vi "PicoScope6000aGetStreamingLatestValues.vi"(0 "handle in":i16=16384, 1 "Polling Delays ms":T1={"Polling holdoff ms"=10, "Polling time ms"=90}, 2 "Buffer and Transfer Settings":T6={"startIndex"=0, "Samples"=1000000, "Down Sample Ratio"=1, "Down-Sample Mode"=2147483648} {"Down-Sample Mode" items=["RAW none"=2147483648, "None"=0, "Aggregate"=1, "Decimate"=2, "Average"=4]; "Down Sample Ratio" step=1; "Samples" format="%_6p"}, 3 "enabled array":i16[](array[numeric])=[1, 1, 0, 0, 0, 0, 0, 0, 0, 0], 5 "Device Info":T3, 7 "Data Pointers In":T4={"Max Buffer Pointers"=[], "Min Buffer Pointers"=[], "StreamingDataInfo"=[[{"Channel"=0, "Down-Sample Mode"=0, "PICO_DATA_TYPE"=enum."PICO_INT16_T", "Samples"=0, "bufferIndex"=0, "startIndex"=0, "overflow"=0}]]}, 9 "Buffer number":i32=1, 11 "error in (no error)":errorcluster) -> (4 "handle out":i16=16384, 8 "Data Pointers Out":T4={"Max Buffer Pointers"=[], "Min Buffer Pointers"=[], "StreamingDataInfo"=[[{"Channel"=0, "Down-Sample Mode"=0, "PICO_DATA_TYPE"=enum."PICO_INT16_T", "Samples"=0, "bufferIndex"=0, "startIndex"=0, "overflow"=0}]]}, 14 "tPicoStreamingDataTriggerInfo":T2, 15 "error out":errorcluster)   [LabVIEW 2010]
doc: "Call ps6000aGetValues to fill a single set of channel buffers."
uses:
  ps6000a.dll
  shared/PicoBuffers.ctl
  shared/Buffer and Transfer Settings.ctl
panel:
  out "No of channels":u64=2
  in  "tPicoStreamingDataInfo":T5={"Channel"=0, "Down-Sample Mode"=2147483648, "PICO_DATA_TYPE"=enum."PICO_INT16_T", "Samples"=0, "bufferIndex"=0, "startIndex"=0, "overflow"=0} {"overflow" step=1 format="%010b"; "Down-Sample Mode" items=["None"=2147483648, "Aggregate"=1, "Decimate"=2, "Average"=4]; "Channel" items=["Channel A"=0, "Channel B"=1, "Channel C"=2, "Channel D"=3, "Channel E"=4, "Channel F"=5, "Channel G"=6, "Channel H"=7, "Port 0"=128, "Port 1"=129, "Trigger AUX"=1001]; "startIndex" step=1}
  in  "Streaming Acquisition Settings":T7={"preTriggerSamples"=0, "postTriggerSamples"=1000000, "Requested sampleInterval"=1.0, "sampleIntervalTimeUnits"=3} {"sampleIntervalTimeUnits" items=["femtoseconds", "picoseconds", "nanoseconds", "microseconds", "millseconds", "seconds"]; "postTriggerSamples" format="%_6p"; "preTriggerSamples" format="%_6p"}
  # "Samples can be equal to or less\nTotal Pre and Post Trigger Samples"
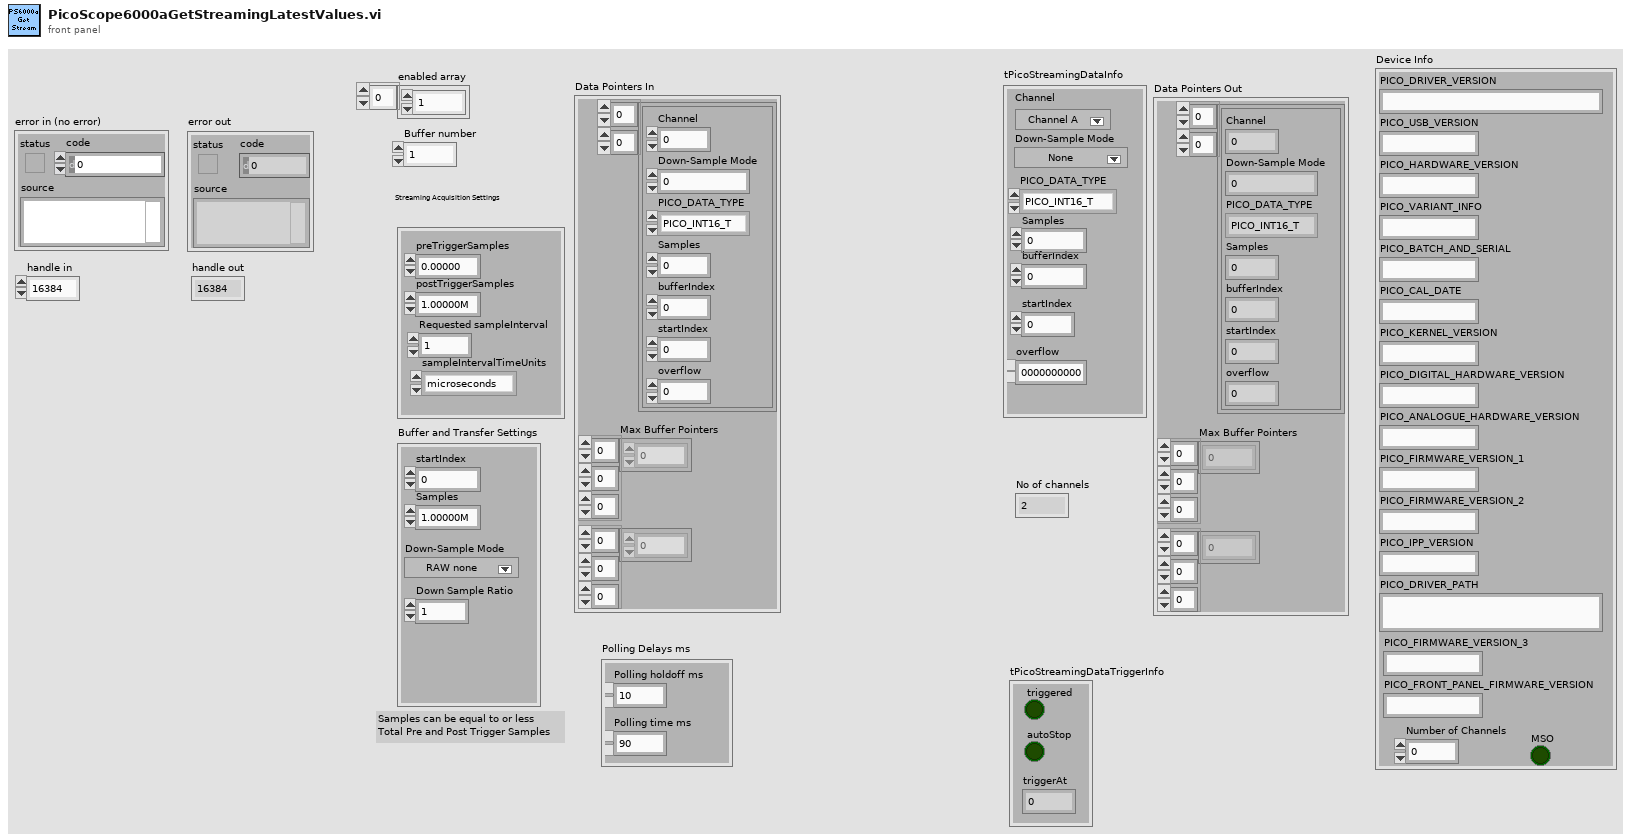
[diagram p1: front panel]
types:
  T1 = cluster{"Polling holdoff ms":u32, "Polling time ms":u32}
  T2 = cluster{"triggerAt":u64, "triggered":bool, "autoStop":bool}
  T3 = cluster{"PICO_DRIVER_VERSION":string, "PICO_USB_VERSION":string, "PICO_HARDWARE_VERSION":string, "PICO_VARIANT_INFO":string, "PICO_BATCH_AND_SERIAL":string, "PICO_CAL_DATE":string, "PICO_KERNEL_VERSION":string, "PICO_DIGITAL_HARDWARE_VERSION":string, "PICO_ANALOGUE_HARDWARE_VERSION":string, "PICO_FIRMWARE_VERSION_1":string, "PICO_FIRMWARE_VERSION_2":string, "PICO_IPP_VERSION":string, "PICO_DRIVER_PATH":string, "PICO_FIRMWARE_VERSION_3":string, "PICO_FRONT_PANEL_FIRMWARE_VERSION":string, "Number of Channels":i16, "MSO":bool}
  T4 = typedef "PicoBuffers.ctl" = cluster{"Max Buffer Pointers":u64[][][], "Min Buffer Pointers":u64[][][], "StreamingDataInfo":cluster{"Channel":u32, "Down-Sample Mode":u32, "PICO_DATA_TYPE":enum32{"PICO_INT8_T", "PICO_INT16_T", "PICO_INT32_T", "PICO_UINT32_T", "PICO_INT64_T", ""}, "Samples":i32, "bufferIndex":u64, "startIndex":i32, "overflow":i16}[][]}
  T5 = cluster{"Channel":u32, "Down-Sample Mode":u32, "PICO_DATA_TYPE":enum32{"PICO_INT8_T", "PICO_INT16_T", "PICO_INT32_T", "PICO_UINT32_T", "PICO_INT64_T", ""}, "Samples":i32, "bufferIndex":u64, "startIndex":i32, "overflow":i16}
  T6 = typedef "Buffer and Transfer Settings.ctl" = cluster{"startIndex":u64, "Samples":u64, "Down Sample Ratio":u64, "Down-Sample Mode":u32}
  T7 = cluster{"preTriggerSamples":u64, "postTriggerSamples":u64, "Requested sampleInterval":dbl, "sampleIntervalTimeUnits":u32}
  T8 = cluster{"triggerAt_":u64, "triggered_":i16, "autoStop_":i16}
  T9 = cluster{"status":bool, "code":u32, "source":string}
  T10 = cluster{"Channel":u32, "Down-Sample Mode":u32, "PICO_DATA_TYPE":enum32{"PICO_INT8_T", "PICO_INT16_T", "PICO_INT32_T", "PICO_UINT32_T", "PICO_INT64_T", ""}, "Samples":i32, "bufferIndex":u64, "startIndex":i32, "overflow":i16}[]
  T11 = cluster{"Channel":u32, "Down-Sample Mode":u32, "PICO_DATA_TYPE":enum32{"PICO_INT8_T", "PICO_INT16_T", "PICO_INT32_T", "PICO_UINT32_T", "PICO_INT64_T", ""}, "Samples":i32, "bufferIndex":u64, "startIndex":i32, "overflow":i16}[][]
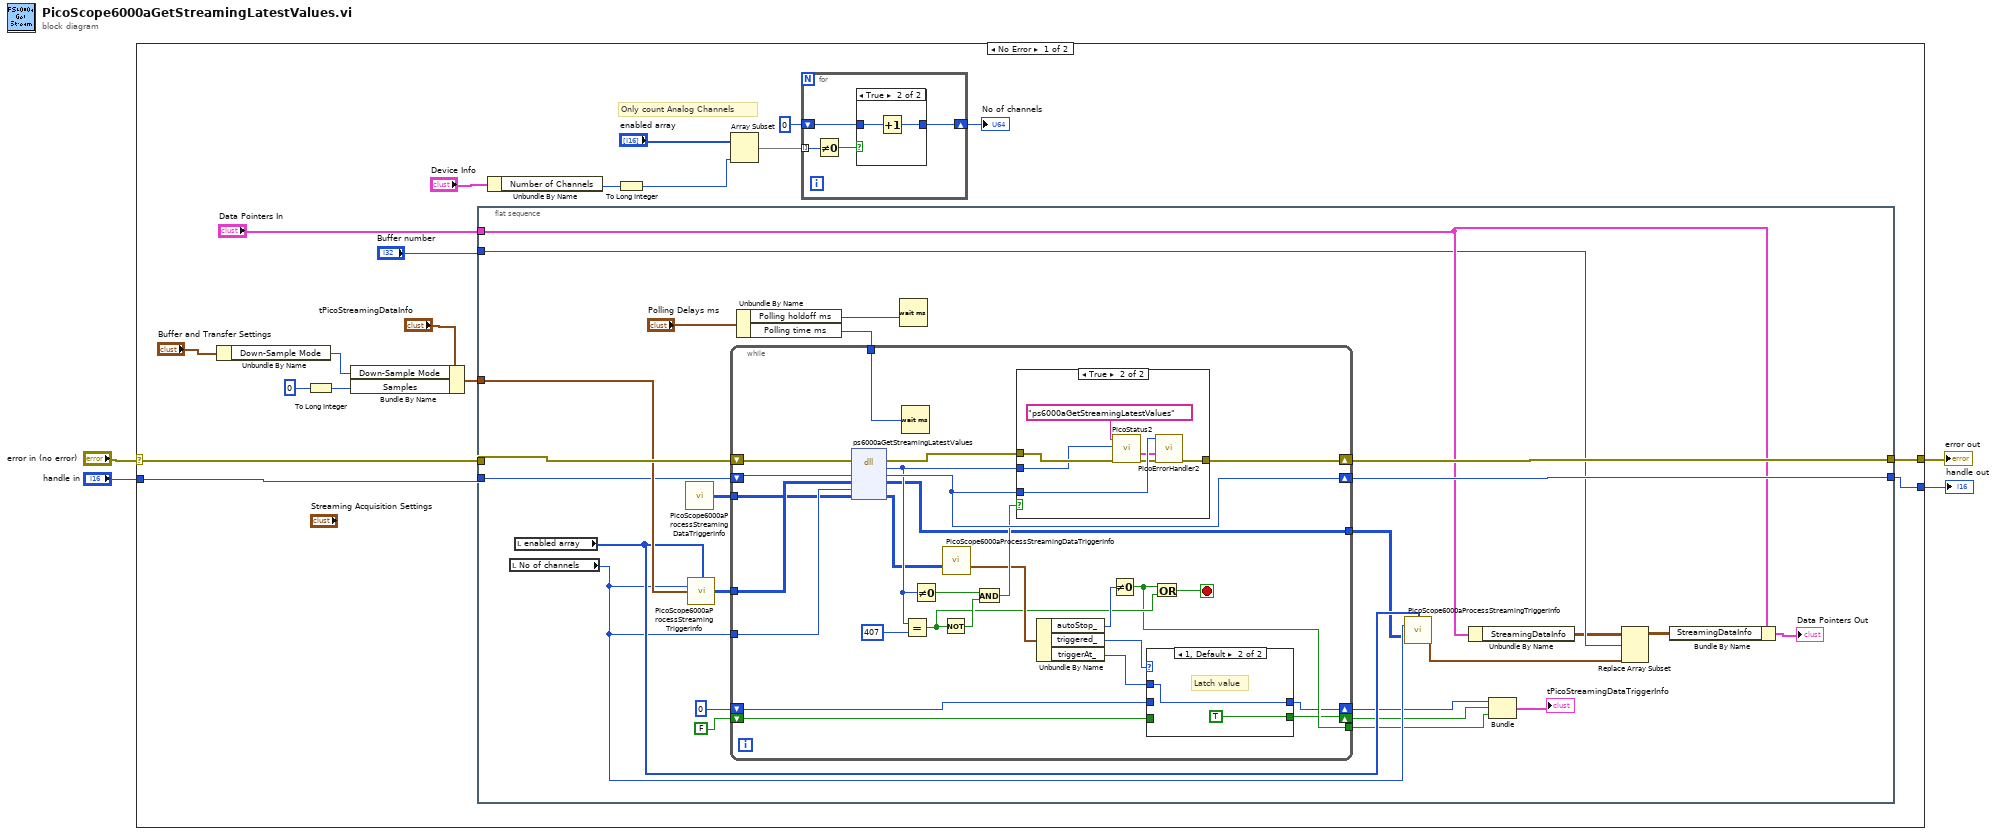
[diagram p0: block diagram]
diagram:
  n1 = case shown="No Error" "error in (no error)" {
    selector: "error in (no error)" -> [w20 w95]
    tunnel: "handle in" -> [w19 w96]
    tunnel: [w23 w96] -> w2
    tunnel: [w21 w95] -> w1
    frame No Error {
      # "Only count Analog Channels"
      n2 = Unbundle By Name("Buffer and Transfer Settings") -> ("Down-Sample Mode"=w15:u32)
      n3 = To Long Integer(number=0) -> (32bit integer=w14:i32)
      n4 = Bundle By Name(cluster="tPicoStreamingDataInfo", "Down-Sample Mode"=w15, "Samples"=w14) -> (w16:T5)
      n5 = flat-sequence {
        tunnel: w20 -> [w55]
        tunnel: w19 -> [w52]
        tunnel: "Buffer number" -> [w45]
        tunnel: w16 -> [w53]
        tunnel: [w51] -> w23
        tunnel: [w54] -> w21
        tunnel: "Data Pointers In" -> [w47]
        frame #0 {
          n6 = local read "No of channels"() -> (w42:u64)
          n7 = local read "enabled array"() -> (w43:i16[])
          n8 = call "PicoScope6000aProcessStreamingDataTriggerInfo.vi"() -> ("C Array for Struture Data Out"=w49:u16[][])  [unwired: 13 in, 2 out]
          n9 = call "PicoScope6000aProcessStreamingTriggerInfo.vi"("enabled array"=w43, "No of C Strutures"=w42, "C Struture define"=w53) -> ("C Array for Struture Data Out"=w48:u16[][])  [unwired: 10 in, 2 out]
          n10 = Unbundle By Name("Polling Delays ms") -> ("Polling holdoff ms"=w38:u32, "Polling time ms"=w37:u32)
          n11 = while {
            shift-right: [w80] -> w54
            shift-left: w55 -> [w82]
            shift-right: [w78] -> w51
            shift-left: w52 -> [w81]
            tunnel: w42 -> [w77]
            tunnel: w48 -> [w76]
            tunnel: w49 -> [w66]
            tunnel: w37 -> [w64]
            tunnel: [w63] -> w41
            tunnel: [w59] -> w33
            shift-right: [w57] -> w31
            shift-left: u64 0 ("triggerAt_") -> [w61]
            shift-right: [w56] -> w32
            shift-left: FALSE ("x = y?") -> [w60]
            stop <- w65 stop-if-true
            n12 = dll-call lib="ps6000a.dll" fn="ps6000aGetStreamingLatestValues" ("ps3000.dll:_ps3000_open_unit@0")(error in=w82, "handle"=w81, "streamingDataInfo"=w76, "nStreamingDataInfos"=w77, "triggerInfo"=w66) -> (error out=w79:errorcluster, "PICO_STATUS"=w74:u32, "handle"=w78:i16, "streamingDataInfo"=w63:u16[][], "triggerInfo"=w70:u16[][])  [unwired: 3 in, 1 out]
            n13 = Wait (ms)(milliseconds to wait=w64) -> ()  [unwired: 1 out]
            n14 = Equal?(x=w74, y=u32 407) -> (x = y?=w67:bool)
            n15 = Not Equal To 0?(x=w74) -> (x != 0?=w72:bool)
            n16 = Not(x=w67) -> (.not. x?=w71:bool)
            n17 = call "PicoScope6000aProcessStreamingDataTriggerInfo.vi"("C Array for Struture Data In"=w70) -> ("tPicoStreamingDataTriggerInfo"=w69:T8)  [unwired: 12 in, 2 out]
            n18 = And(x=w72, y=w71) -> (x .and. y?=w73:bool)
            n19 = case shown="True" w73 {
              tunnel: w78 -> [_ w94]
              tunnel: [w87 w93] -> w80
              tunnel: w74 -> [_ w88]
              tunnel: w79 -> [w87 w90]
              frame False {
              }
              frame True {
                n20 = call "PicoStatus2.vi"("PICO source"="ps6000aGetStreamingLatestValues" ("source"), "Error in"=w90, "PICO STATUS"=w88) -> ("error out"=w92:errorcluster, "PICO_STATUS out"=w89:T9)  [unwired: 5 in]
                n21 = call "PicoErrorHandler2.vi"("error in (no error)"=w92, "PICO_STATUS in"=w89, "handle In"=w94) -> ("error out"=w93:errorcluster)  [unwired: 8 in]
              }
            }
            n22 = Unbundle By Name(w69) -> ("autoStop_"=w68:i16, "triggered_"=w62:i16, "triggerAt_"=w58:u64)
            n23 = Not Equal To 0?(x=w68) -> (x != 0?=w59:bool)
            n24 = case shown="1, Default" w62 {
              tunnel: w61 -> [w83 _]
              tunnel: [w83 w85] -> w57
              tunnel: w60 -> [w84 _]
              tunnel: [w84 TRUE ("x = y?")] -> w56
              tunnel: w58 -> [_ w85]
              frame 0 {
              }
              frame 1, Default {
                # "Latch value"
              }
            }
            n25 = Or(x=w59, y=w67) -> (x .or. y?=w65:bool)
          }
          n26 = Wait (ms)(milliseconds to wait=w38) -> ()  [unwired: 1 out]
          n27 = call "PicoScope6000aProcessStreamingTriggerInfo.vi"("enabled array"=w43, "No of C Strutures"=w42, "C Array for Struture Data In"=w41) -> ("Array of Clusters"=w40:T10)  [unwired: 10 in, 2 out]
          n28 = Unbundle By Name(w47) -> ("StreamingDataInfo"=w44:T11)
          n29 = Bundle("triggerAt_"=w31, "x = y?"=w32, w33) -> (→"tPicoStreamingDataTriggerInfo":cluster{"triggerAt_":u64, "x = y?":bool, bool})  [unwired: 1 in]
          n30 = Replace Array Subset(array=w44, new element=w40, index (row)=w45) -> (w46:T11)  [unwired: 1 in]
          n31 = Bundle By Name(cluster=w47, "StreamingDataInfo"=w46) -> (→"Data Pointers Out":T4)
        }
      }
      n32 = Unbundle By Name("Device Info") -> ("Number of Channels"=w11:i16)
      n33 = To Long Integer(number=w11) -> (32bit integer=w9:i32)
      n34 = Array Subset(array="enabled array", length=w9) -> (w5:i16[])  [unwired: 1 in]
      n35 = for {
        shift-right: [w27] -> w8
        shift-left: u64 0 -> [w26]
        tunnel: w5 -> [w25] mode=indexing
        n36 = Not Equal To 0?(x=w25) -> (x != 0?=w24:bool)
        n37 = case shown="True" w24 {
          tunnel: [w28 w30] -> w27
          tunnel: w26 -> [w28 w29]
          frame False {
          }
          frame True {
            n38 = Increment(x=w29) -> (x+1=w30:u64)
          }
        }
      }
      "No of channels" <- w8
    }
    frame Error {
    }
  }
  "handle out" <- w2
  "error out" <- w1
